vi "Read TrayStatus.vi"(8 "error in (no error)":errorcluster, 10 "F1/T2":bool, 11 "Station Action in":refnum<class "Station Action.lvclass">) -> (0 "error out":errorcluster, 1 "Arr_TrayST":bool[][](array[boolean]), 2 "Arr_Tray":cluster{"X":sgl, "Y":sgl}[][](array[cluster]), 3 "Station Action out":refnum<class "Station Action.lvclass">)   [LabVIEW 2019, in "Station Action.lvclass"]
uses:
  Station Action.lvclass
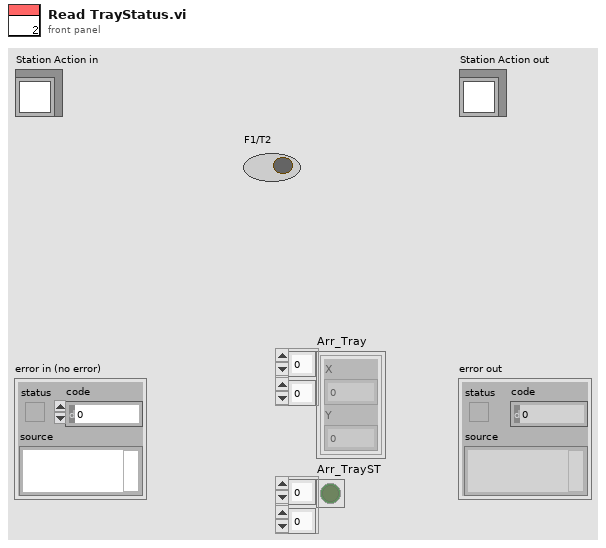
[diagram p1: front panel]
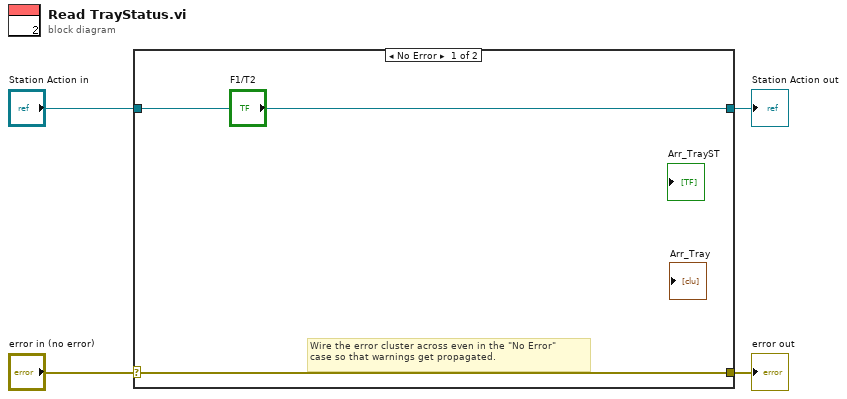
[diagram p0: block diagram]
diagram:
  n1 = case shown="No Error" "error in (no error)" {
    selector: "error in (no error)" -> [w5 w8]
    tunnel: [w5 w8] -> w3
    tunnel: [w6 w7] -> w1
    tunnel: "Station Action in" -> [w6 w7]
    frame No Error {
      # "Wire the error cluster across even in the \"No Error\"\ncase so that warnings get propagated."
    }
    frame Error {
    }
  }
  "error out" <- w3
  "Station Action out" <- w1
